vi "Insert Element In 2D Array (DBL).vi"(8 "Input Array":dbl[][](array[numeric]), 9 "column":dbl, 11 "Element":dbl) -> (2 "Output Array":dbl[][](array[numeric]))   [LabVIEW 2014]
doc: "Inserts a single element in a 2D array.\nThis cannot be accomplished with Insert Into Array or Replay Array Subset."
panel:
  out "output array":dbl[](array[numeric])
  out "subarray":dbl[](array[numeric])
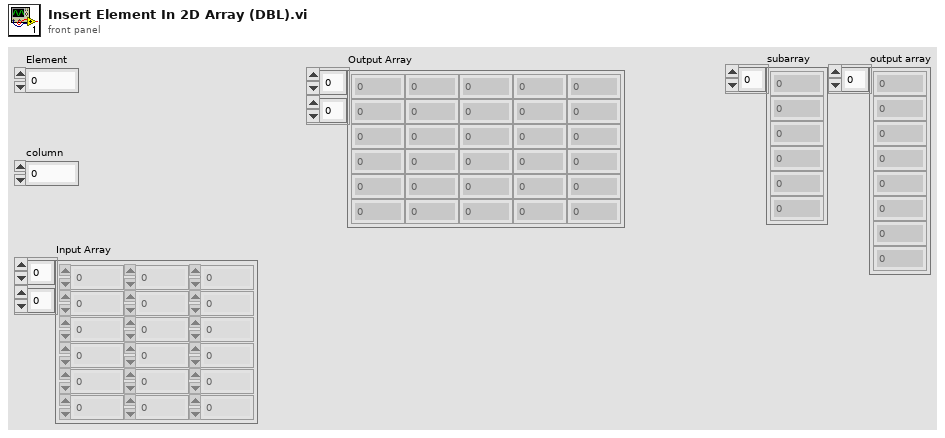
[diagram p1: front panel]
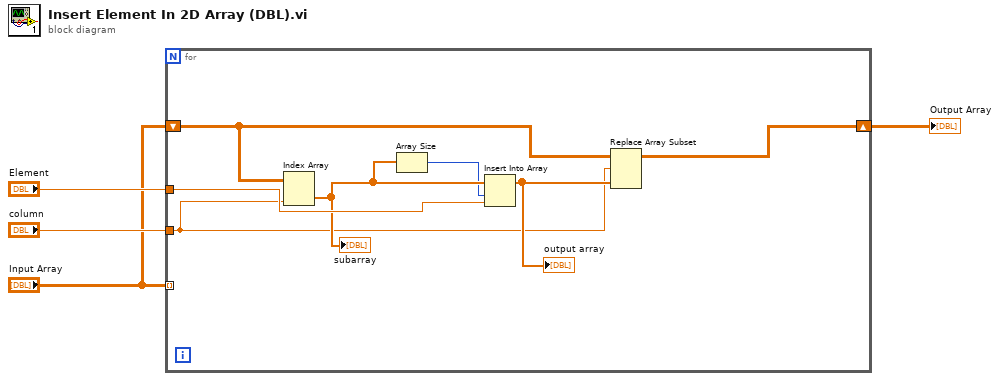
[diagram p0: block diagram]
diagram:
  n1 = for {
    tunnel: "Input Array" -> [_] mode=indexing
    tunnel: "Element" -> [w11]
    tunnel: "column" -> [w5]
    shift-right: [w8] -> w1
    shift-left: "Input Array" -> [w10]
    n2 = Index Array(array=w10, index (col)=w5) -> (element=w7:dbl[])  [unwired: 1 in]
    "subarray" <- w7
    n3 = Array Size(array=w7) -> (size(s)=w6:i32)
    n4 = Insert Into Array(array=w7, index=w6, new element=w11) -> (w9:dbl[])
    "output array" <- w9
    n5 = Replace Array Subset(array=w10, new element=w9, index (row)=w5) -> (w8:dbl[][])  [unwired: 1 in]
  }
  "Output Array" <- w1
